vi "Save Data (Index).vi"(0 "Filepath":path, 2 "DataRowIndex":i32, 3 "Data":string[](array[string]), 7 "xlRefs":T1, 11 "Error In":errorcluster) -> (15 "Error Out":errorcluster)   [LabVIEW 2013]
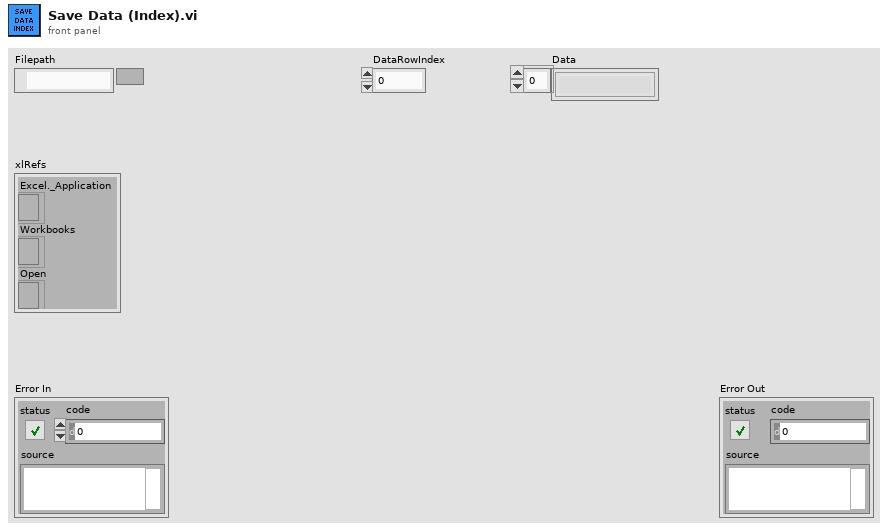
[diagram p1: front panel]
types:
  T1 = cluster{"Excel._Application":refnum<k7>, "Workbooks":refnum<k7>, "Open":refnum<k7>}
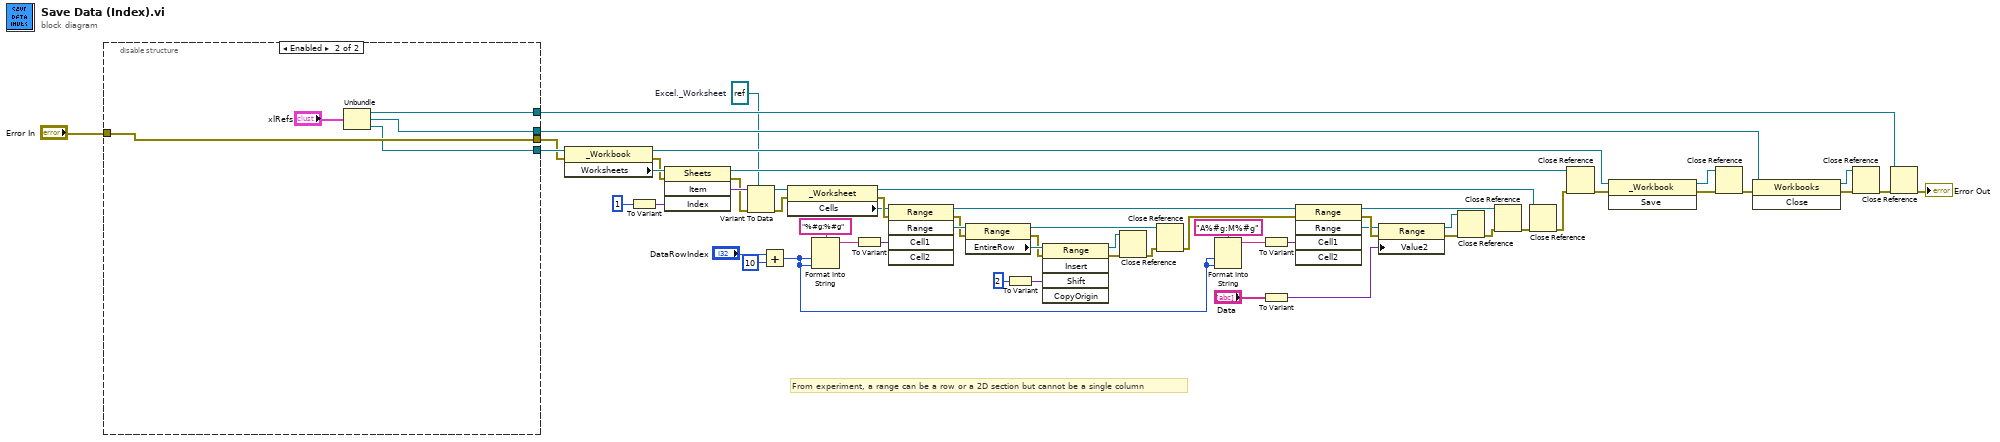
[diagram p0: block diagram]
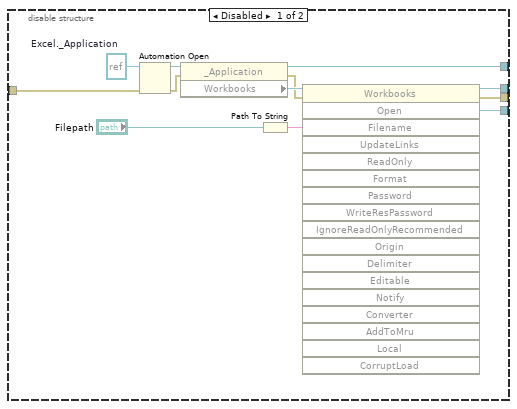
[diagram p2: hidden frame]
diagram:
  w44 = refnum<k7> refnum  # Excel._Worksheet
  # "From experiment, a range can be a row or a 2D section but cannot be a single column"
  n1 = disable-structure shown="Enabled" {
    disable-tunnel: [w66 w71] -> w58
    disable-tunnel: [w65 w72] -> w56
    disable-tunnel: [w63 w73] -> w53
    disable-tunnel: [w62 w75] -> w52
    disable-tunnel: "Error In" -> [w60 w75]
    frame Disabled {
      w67 = refnum<k7> refnum  # Excel._Application
      n2 = Automation Open(error in (no error)=w60, Automation Refnum=w67) -> (Automation Refnum=w68:refnum<k7>, error out=w69:errorcluster)  [unwired: 2 in]
      n3 = property class="_Application"(reference=w68, error in=w69) -> (reference out=w63:refnum<k7>, error out=w64:errorcluster, "Workbooks"=w70:refnum<k7>)
      n4 = Path To String(path="Filepath") -> (string=w61:string)
      n5 = invoke class="Workbooks" method="Open"(reference=w70, error in=w64, "Filename"=w61) -> (reference out=w65:refnum<k7>, error out=w62:errorcluster, "Open"=w66:refnum<k7>)  [unwired: 15 in, 15 out]
    }
    frame Enabled {
      n6 = Unbundle("xlRefs") -> ("Excel._Application"=w73:refnum<k7>, "Workbooks"=w72:refnum<k7>, "Open"=w71:refnum<k7>)
    }
  }
  n7 = property class="_Workbook"(reference=w58, error in=w52) -> (reference out=w47:refnum<k7>, error out=w1:errorcluster, "Worksheets"=w2:refnum<k7>)
  n8 = To Variant(anything=1) -> (Variant=w39:variant)
  n9 = invoke class="Sheets" method="Item"(reference=w2, error in=w1, "Index"=w39) -> (reference out=w45:refnum<k7>, error out=w37:errorcluster, "Item"=w38:variant)  [unwired: 1 in, 1 out]
  n10 = Variant To Data(error in=w37, type=w44, Variant=w38) -> (data=w36:refnum<k7>, error out=w35:errorcluster)
  n11 = Add(x="DataRowIndex", y=10) -> (x+y=w11:i32)
  n12 = property class="_Worksheet"(reference=w36, error in=w35) -> (reference out=w33:refnum<k7>, error out=w18:errorcluster, "Cells"=w17:refnum<k7>)
  n13 = Format Into String(format string="%#g:%#g", w11, w11) -> (resulting string=w16:string)  [unwired: 2 in, 1 out]
  n14 = To Variant(anything=w16) -> (Variant=w19:variant)
  n15 = invoke class="Range" method="Range"(reference=w17, error in=w18, "Cell1"=w19) -> (reference out=w10:refnum<k7>, error out=w9:errorcluster, "Range"=w15:refnum<k7>)  [unwired: 2 in, 2 out]
  n16 = property class="Range"(reference=w15, error in=w9) -> (reference out=w5:refnum<k7>, error out=w8:errorcluster, "EntireRow"=w14:refnum<k7>)
  n17 = To Variant(anything=2) -> (Variant=w13:variant)
  n18 = invoke class="Range" method="Insert"(reference=w14, error in=w8, "Shift"=w13) -> (reference out=w6:refnum<k7>, error out=w7:errorcluster)  [unwired: 2 in, 3 out]
  n19 = Close Reference(reference=w6, error in (no error)=w7) -> (error out=w4:errorcluster)
  n20 = Close Reference(reference=w5, error in (no error)=w4) -> (error out=w3:errorcluster)
  n21 = Format Into String(format string="A%#g:M%#g", w11, w11) -> (resulting string=w22:string)  [unwired: 2 in, 1 out]
  n22 = To Variant(anything=w22) -> (Variant=w27:variant)
  n23 = To Variant(anything="Data") -> (Variant=w25:variant)
  n24 = invoke class="Range" method="Range"(reference=w10, error in=w3, "Cell1"=w27) -> (reference out=w32:refnum<k7>, error out=w26:errorcluster, "Range"=w21:refnum<k7>)  [unwired: 2 in, 2 out]
  n25 = property class="Range"(reference=w21, error in=w26, "Value2"=w25) -> (reference out=w24:refnum<k7>, error out=w23:errorcluster)
  n26 = Close Reference(reference=w24, error in (no error)=w23) -> (error out=w31:errorcluster)
  n27 = Close Reference(reference=w32, error in (no error)=w31) -> (error out=w34:errorcluster)
  n28 = Close Reference(reference=w33, error in (no error)=w34) -> (error out=w46:errorcluster)
  n29 = Close Reference(reference=w45, error in (no error)=w46) -> (error out=w51:errorcluster)
  n30 = invoke class="_Workbook" method="Save"(reference=w47, error in=w51) -> (reference out=w48:refnum<k7>, error out=w49:errorcluster)  [unwired: 1 in, 1 out]
  n31 = Close Reference(reference=w48, error in (no error)=w49) -> (error out=w50:errorcluster)
  n32 = invoke class="Workbooks" method="Close"(reference=w56, error in=w50) -> (reference out=w55:refnum<k7>, error out=w54:errorcluster)  [unwired: 1 in, 1 out]
  n33 = Close Reference(reference=w55, error in (no error)=w54) -> (error out=w57:errorcluster)
  n34 = Close Reference(reference=w53, error in (no error)=w57) -> (error out=→"Error Out":errorcluster)
